vi "Skew Accumulator (SubVI).vi"(0 "New Skew Value":dbl, 5 "Reset Skew Graph":bool, 7 "xIncrement":dbl, 9 "Triggered?":bool) -> (4 "Skew Histogram":T1(graph), 6 "Skew vs. Time":waveform(dbl), 8 "Skew Max":dbl format="%#_5p", 10 "Skew Min":dbl format="%#_5p")   [LabVIEW 2022 SP3]
uses:
  <vilib>/Analysis/NI_AALBase.lvlib
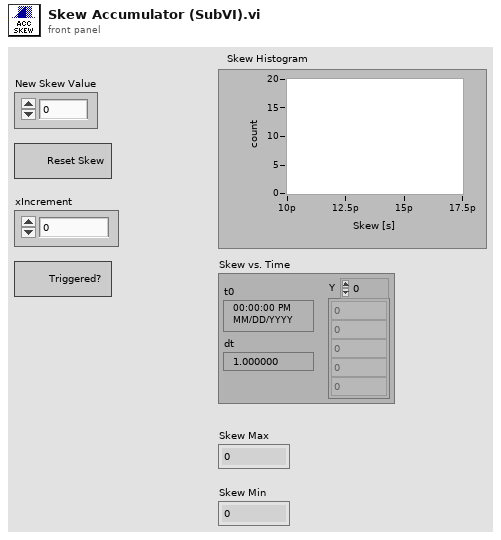
[diagram p1: front panel]
types:
  T1 = cluster{"X Values":dbl[], "Histogram: h(x)":i32[]}
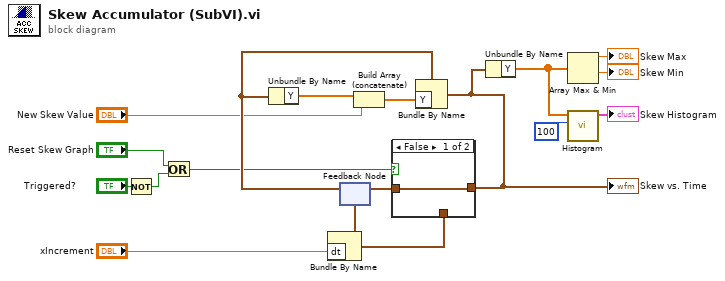
[diagram p0: block diagram]
diagram:
  n1 = Not(x="Triggered?") -> (.not. x?=w10:bool)
  n2 = Or(x="Reset Skew Graph", y=w10) -> (x .or. y?=w8:bool)
  n3 = Bundle By Name("dt"="xIncrement") -> (w17:waveform(dbl))  [unwired: 1 in]
  n4 = feedback #1(w17) -> (w15:waveform(dbl))
  n5 = Unbundle By Name(w15) -> ("Y"=w14:dbl[])
  n6 = Build Array (concatenate)(w14, "New Skew Value") -> (w3:dbl[])
  n7 = Bundle By Name(cluster=w15, "Y"=w3) -> (w2:waveform(dbl))
  "Skew vs. Time" <- w2
  n8 = case shown="False" w8 {
    tunnel: w2 -> [w18 _]
    tunnel: [w18 w19] -> w16
    tunnel: w17 -> [_ w19]
    frame False {
    }
    frame True {
    }
  }
  n9 = feedback-in #1(w16) -> ()
  n10 = Unbundle By Name(w2) -> ("Y"=w1:dbl[])
  n11 = Array Max & Min(array=w1) -> (max value=→"Skew Max":dbl, min value=→"Skew Min":dbl)  [unwired: 2 out]
  n12 = call <vilib>:"Histogram.vi"("intervals"=100, "X"=w1) -> ("Histogram Graph"=→"Skew Histogram":T1)  [unwired: 6 in, 3 out]
